vi "Camera_Read Settings.vi"(8 "Error":errorcluster, 11 "CameraDevRef":T6) -> (0 "Error Out":errorcluster, 2 "Camera Settings":T1 {"Saturation" min=0 max=100 step=1; "Sharpness" min=0 max=100 step=1; "Brightness" min=0 max=100 step=1; "Exposure (%)" min=0.0 max=100.0 step=1.0}, 3 "CameraDevRef Out":T6)   [LabVIEW 2017, in "VisionSystem.lvlib"]
uses:
  VisionSystem.lvlib
  <vilib>/Rock Robotics/WPI/Camera/WPI_CameraDevRef.ctl
  TypeDefs/Cluster_Camera Settings.ctl
  <vilib>/Rock Robotics/WPI/Camera/WPI_CameraImageSize.ctl
  <vilib>/Rock Robotics/WPI/Camera/WPI_CameraFrameRate.ctl
  <vilib>/Rock Robotics/WPI/Camera/WPI_CameraWhite Balance Values.ctl
  <vilib>/Rock Robotics/WPI/Camera/WPI_CameraExposure Values.ctl
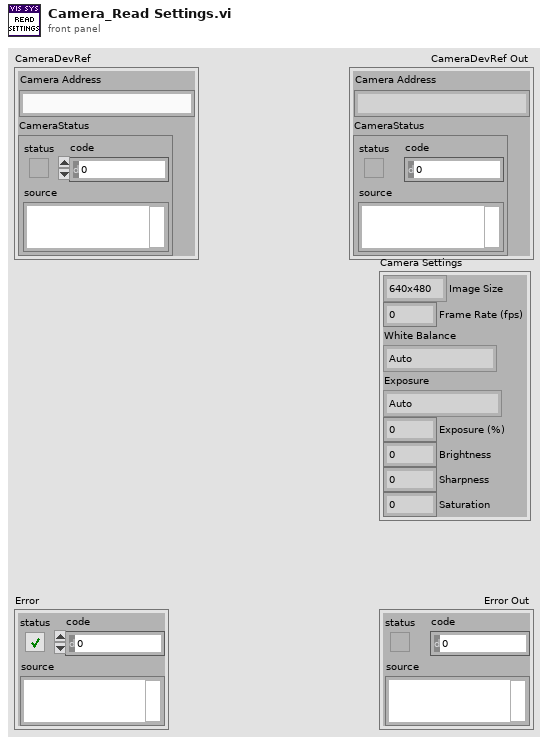
[diagram p1: front panel]
types:
  T1 = typedef "Cluster_Camera Settings.ctl" = cluster{"Image Size":T2, "Frame Rate (fps)":T3, "White Balance":T4, "Exposure":T5, "Exposure (%)":dbl, "Brightness":i32, "Sharpness":i32, "Saturation":i32}
  T2 = typedef "WPI_CameraImageSize.ctl" = enum16{"640x480", "320x240", "160x120", "Custom"}
  T3 = typedef "WPI_CameraFrameRate.ctl" = u32
  T4 = typedef "WPI_CameraWhite Balance Values.ctl" = enum16{"Auto", "Fixed indoor", "Fixed outdoor 1", "Fixed outdoor 2", "Fixed fluorescent 1", "Fixed fluorescent 2", "Hold current", "Custom"}
  T5 = typedef "WPI_CameraExposure Values.ctl" = enum16{"Auto", "Flicker-free 50 Hz", "Flicker-free 60 Hz", "Hold current", "Custom"}
  T6 = typedef "WPI_CameraDevRef.ctl" = cluster{"Camera Address":string, "CameraStatus":errorcluster}
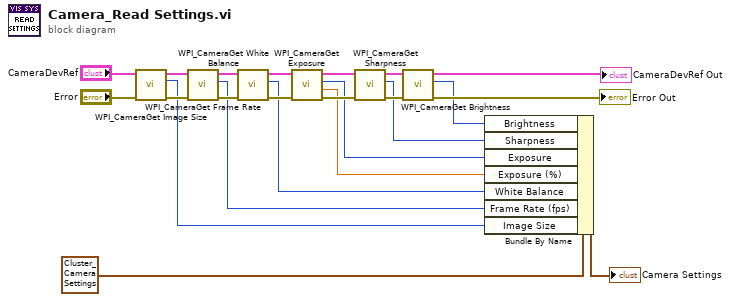
[diagram p0: block diagram]
diagram:
  n1 = call <vilib>:"WPI_CameraGet Image Size.vi"("error in (no error)"="Error", "CameraDevRef"="CameraDevRef") -> ("error out"=w15:errorcluster, "Image Size"=w2:T2, "CameraDevRef Out"=w18:T6)  [unwired: 6 in, 1 out]
  n2 = call <vilib>:"WPI_CameraGet Frame Rate.vi"("error in (no error)"=w15, "CameraDevRef"=w18) -> ("error out"=w14:errorcluster, "Frame Rate (fps)"=w3:T3, "CameraDevRef Out"=w20:T6)  [unwired: 7 in]
  n3 = call <vilib>:"WPI_CameraGet White Balance.vi"("error in (no error)"=w14, "CameraDevRef"=w20) -> ("error out"=w13:errorcluster, "White Balance"=w4:T4, "CameraDevRef Out"=w19:T6)  [unwired: 6 in, 1 out]
  n4 = call <vilib>:"WPI_CameraGet Exposure.vi"("error in (no error)"=w13, "CameraDevRef"=w19) -> ("error out"=w12:errorcluster, "Exposure (%)"=w5:dbl, "Exposure"=w6:T5, "CameraDevRef Out"=w22:T6)  [unwired: 6 in]
  n5 = call <vilib>:"WPI_CameraGet Sharpness.vi"("error in (no error)"=w12, "CameraDevRef"=w22) -> ("error out"=w11:errorcluster, "Sharpness"=w1:i32, "CameraDevRef Out"=w21:T6)  [unwired: 7 in]
  n6 = call <vilib>:"WPI_CameraGet Brightness.vi"("error in (no error)"=w11, "CameraDevRef"=w21) -> ("error out"=→"Error Out":errorcluster, "Brightness"=w7:i32, "CameraDevRef Out"=→"CameraDevRef Out":T6)  [unwired: 7 in]
  n7 = Bundle By Name(cluster=T1 {"Image Size"=enum."640x480", "Frame Rate (fps)"=0, "White Balance"=enum."Auto", "Exposure"=enum."Auto", "Exposure (%)"=0.0, "Brightness"=0, "Sharpness"=0, "Saturation"=0} ("Camera Settings"), "Brightness"=w7, "Sharpness"=w1, "Exposure"=w6, "Exposure (%)"=w5, "White Balance"=w4, "Frame Rate (fps)"=w3, "Image Size"=w2) -> (→"Camera Settings":T1)
